vi "运维调试_采配水V2.vi"() -> ()   [LabVIEW 2016, in "PLC.lvlib"]
uses:
  PLC.lvlib
  <vilib>/Plasmionique/MB Master/MB_Master/MB_Master.lvclass
  <vilib>/Utility/miscctls.llb/LVPointTypeDef.ctl
  <vilib>/Plasmionique/MB Master/MB_Master_Serial/MB_Master_Serial.lvclass
  D:/Program Files (x86)/National Instruments/LabVIEW 2016/vi.lib/Plasmionique/MB Master/MB_Master/MB_Master.lvclass
  <vilib>/Instr/_visa.llb/VISA Configure Serial Port (Instr).vi
  <vilib>/Plasmionique/MB Master/MB Master.lvlib
panel:
  out "Registers":u16[](array[numeric])
  out "R118":i16 caption="多参数沉淀时间"
  in  "看门狗启用":bool
  out "R117":i16 caption="看门狗设置值"
  out "R33":i16 caption="看门狗计时器"
  in  "更新程序":bool
  in  "R116":i16(ring) caption="储水水体选择" items=["自来水", "采水泵"]
  out "当前启动泵号":u16(ring) items=["1号水样泵", "2号水样泵"]
  out "R113":i16 caption="储水时间设定"
  out "R25":i16
  in  "V14NC":bool
  out "R24":i16
  in  "V14NO":bool
  out "X2":bool caption="X1"
  out "采配水版本号":string
  out "R23":i16 caption="清洗频次计数"
  out "R112":i16 caption="清洗频次设定"
  out "R22":i16
  in  "V13NC":bool
  out "R111":i16 caption="排液时间"
  out "通讯故障":bool
  out "R21":i16
  in  "V13NO":bool
  out "R20":i16
  in  "M1-2":bool
  in  "潜水泵工作模式":u16(ring) items=["泵1单泵单管路", "泵2单泵单管路", "潜水泵双泵双管路", "自吸泵双泵双管路"]
  out "X11":bool caption="废液报警"
  out "X10":bool caption="自来水检测"
  out "X9":bool caption="泵2过载报警"
  out "X8":bool caption="泵1过载报警"
  out "X7":bool caption="断电检测"
  out "X6":bool caption="开门检测"
  out "X5":bool caption="烟雾检测"
  out "X4":bool caption="漏水检测"
  out "X3":bool caption="进样检测"
  out "X1":bool
  out "X0":bool caption="采样池液位开关"
  out "R109":i16 caption="配水时间"
  out "集成报警信息":string
  out "R108":i16 caption="自来水报警"
  out "R107":i16 caption="采水池液位报警设置"
  out "R106":i16 caption="进样超时设置"
  out "R105":i16 caption="二级清洗时间"
  out "R104":i16 caption="一级清洗时间"
  out "R103":i16 caption="外部管路清洗时间"
  out "R102":i16 caption="静置沉淀时间"
  out "R101":i16 caption="内部管路润洗时间"
  out "R100":i16 caption="外部管路润洗时间"
  out "R2":i16
  out "R1":i16
  out "多列列表框":i32(listbox)
  out "R19":i16
  in  "V6":bool
  out "R18":i16
  in  "V5":bool
  out "R17":i16
  in  "V4":bool
  out "R16":i16
  in  "V3":bool
  out "R15":i16
  in  "V2":bool
  out "R14":i16
  in  "M2":bool
  out "R13":i16
  in  "V1":bool
  out "R12":i16
  in  "M1-1":bool
  in  "返回":bool
  in  "参数设置":bool
  in  "单步启动":bool
  in  "启动":bool
  in  "停止":bool
  # "看门狗设置"
  # "S"
  # "S"
  # "S"
  # "S"
  # "次"
  # "次"
  # "S"
  # "S"
  # "S"
  # "S"
  # "S"
  # "S"
  # "S"
  # "S"
  # "S"
  # "S"
  # "S"
  # "单步计时："
  # "s"
  # "流程计时："
  # "s"
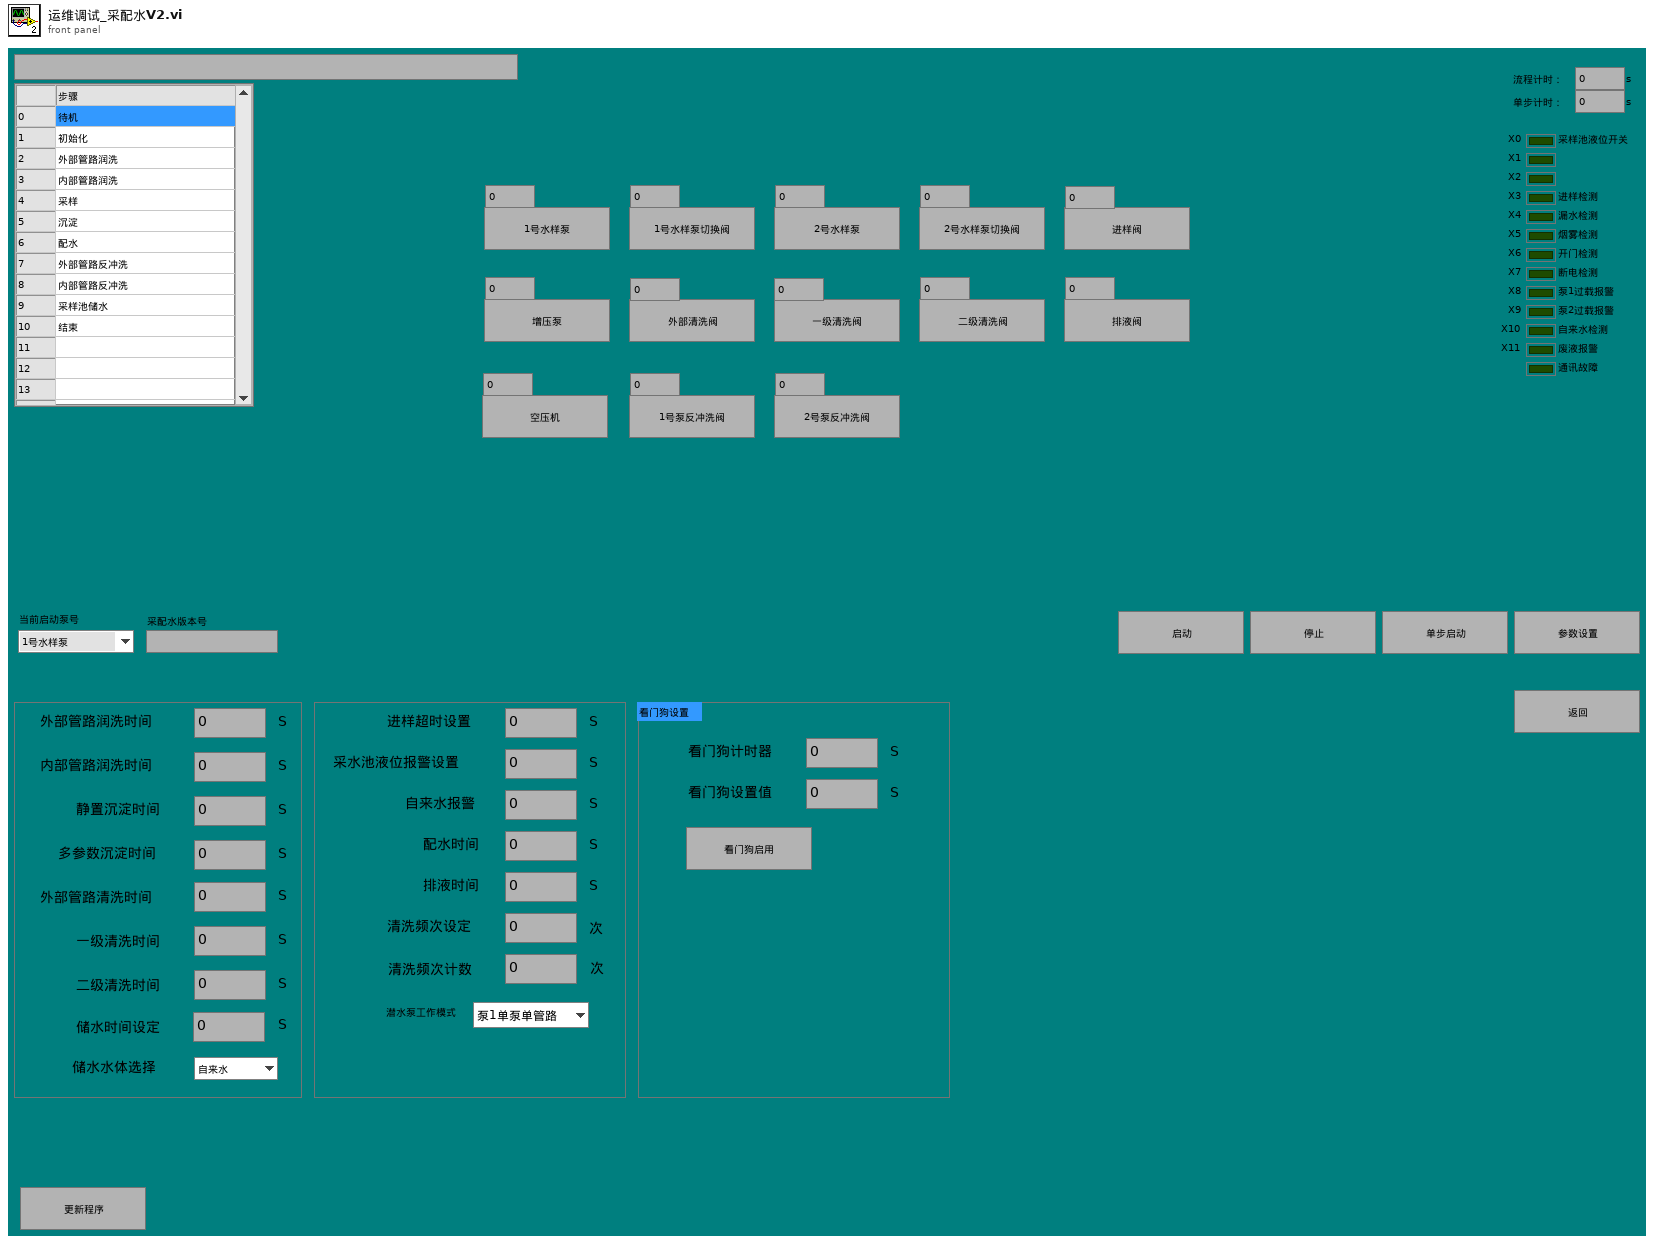
[diagram p1: front panel]
types:
  T1 = typedef "参数.ctl" = cluster{"测试模式":enum16{"水样测试", "平行样测试", "集成干预测试", "加标回收"}, "参数启用":T2}
  T2 = typedef "启动参数.ctl" = cluster{"氨氮":bool, "总磷":bool, "总氮":bool, "多参数":bool, "CODmn":bool, "CODCr":bool, "氟化物":bool, "超标留样启用":bool}
  T3 = typedef "LVPointTypeDef.ctl" = cluster{"Horizontal":i16, "Vertical":i16}
  T4 = cluster{"命令":string, "数据":cluster{"starting address":u16, "holding register value":u16}}
  T5 = cluster{"命令":string, cluster{"starting address":u16, "holding register value":u16}}
  T6 = cluster{"命令":string, "数据":cluster{"starting address":u16, "holding register values":u16[]}}
  T7 = cluster{"命令":string, "data":cluster{"starting address":u16, "coil values":bool[]}}
  T8 = cluster{"测试模式":enum16{"水样测试", "平行样测试", "集成干预测试", "加标回收"}, "参数启用":T2}
  T9 = cluster{"R0":i16, "R1":i16, "R2":i16, "R3":i16, "R4":i16, "R5":i16, "R6":i16, "R7":i16, "R8":i16, "R9":i16, "R10":i16, "R11":i16, "R12":i16, "R13":i16, "R14":i16, "R15":i16, "R16":i16, "R17":i16, "R18":i16, "R19":i16, "R20":i16, "R21":i16, "R22":i16, "R23":i16, "R24":i16, "R25":i16, "R26":i16, "R27":i16, "R28":i16, "R29":i16, "R30":i16, "R31":i16, "R32":i16, "R33":i16, "R34":i16, "R35":i16, "R36":i16, "R37":i16, "R38":i16, "R39":i16, "R40":i16, "R41":i16, "R42":i16, "R43":i16, "R44":i16, "R45":i16, "R46":i16, "R47":i16, "R48":i16, "R49":i16, "R50":i16, "R51":i16, "R52":i16, "R53":i16, "R54":i16, "R55":i16, "R56":i16, "R57":i16, "R58":i16, "R59":i16, "R60":i16, "R61":i16, "R62":i16, "R63":i16, "R64":i16, "R65":i16, "R66":i16, "R67":i16, "R68":i16, "R69":i16, "R70":i16, "R71":i16, "R72":i16, "R73":i16, "R74":i16, "R75":i16, "R76":i16, "R77":i16, "R78":i16, "R79":i16}
  T10 = cluster{"R100":i16, "R101":i16, "R102":i16, "R103":i16, "R104":i16, "R105":i16, "R106":i16, "R107":i16, "R108":i16, "R109":i16, "R110":i16, "R111":i16, "R112":i16, "R113":i16, "R114":i16, "R115":i16, "R116":i16, "R117":i16, "R118":i16, "R119":i16, "R120":i16, "R121":i16, "R122":i16, "R123":i16, "R124":i16, "R125":i16, "R126":i16, "R127":i16, "R128":i16, "R129":i16, "R130":i16, "R131":i16, "R132":i16, "R133":i16}
  T11 = cluster{"seconds since 1Jan1904":timestamp, "table输入":string, string, "table输入":string}
  T12 = cluster{"baud rate (bps)":u32, "stop bits":u16, "parity":u16, "flow control":u16, "timeout":u32, "retries":i32}
  T13 = cluster{"starting address":u16, "holding register values":u16[]}
  T14 = cluster{"starting address":u16, "holding register value":u16}
  T15 = cluster{"starting address":u16, "coil values":bool[]}
  T16 = cluster{"Registers[0]":u16, "Registers[1]":u16, "Registers[2]":u16, "Registers[3]":u16, "Registers[4]":u16, "Registers[5]":u16, "Registers[6]":u16, "Registers[7]":u16, "Registers[8]":u16, "Registers[9]":u16, "Registers[10]":u16, "Registers[11]":u16, "Registers[12]":u16, "Registers[13]":u16, "Registers[14]":u16, "Registers[15]":u16, "Registers[16]":u16, "Registers[17]":u16, "Registers[18]":u16, "Registers[19]":u16, "Registers[20]":u16, "Registers[21]":u16, "Registers[22]":u16, "Registers[23]":u16, "Registers[24]":u16, "Registers[25]":u16, "Registers[26]":u16, "Registers[27]":u16, "Registers[28]":u16, "Registers[29]":u16, "Registers[30]":u16, "Registers[31]":u16, "Registers[32]":u16, "Registers[33]":u16, "Registers[34]":u16, "Registers[35]":u16, "Registers[36]":u16, "Registers[37]":u16, "Registers[38]":u16, "Registers[39]":u16, "Registers[40]":u16, "Registers[41]":u16, "Registers[42]":u16, "Registers[43]":u16, "Registers[44]":u16, "Registers[45]":u16, "Registers[46]":u16, "Registers[47]":u16, "Registers[48]":u16, "Registers[49]":u16, "Registers[50]":u16, "Registers[51]":u16, "Registers[52]":u16, "Registers[53]":u16, "Registers[54]":u16, "Registers[55]":u16, "Registers[56]":u16, "Registers[57]":u16, "Registers[58]":u16, "Registers[59]":u16, "Registers[60]":u16, "Registers[61]":u16, "Registers[62]":u16, "Registers[63]":u16, "Registers[64]":u16, "Registers[65]":u16, "Registers[66]":u16, "Registers[67]":u16, "Registers[68]":u16, "Registers[69]":u16, "Registers[70]":u16, "Registers[71]":u16, "Registers[72]":u16, "Registers[73]":u16, "Registers[74]":u16, "Registers[75]":u16, "Registers[76]":u16, "Registers[77]":u16, "Registers[78]":u16, "Registers[79]":u16}
  T17 = cluster{"Registers[0]":u16, "Registers[1]":u16, "Registers[2]":u16, "Registers[3]":u16, "Registers[4]":u16, "Registers[5]":u16}
  T18 = cluster{"Registers[0]":u16, "Registers[1]":u16, "Registers[2]":u16, "Registers[3]":u16, "Registers[4]":u16, "Registers[5]":u16, "Registers[6]":u16, "Registers[7]":u16, "Registers[8]":u16, "Registers[9]":u16, "Registers[10]":u16, "Registers[11]":u16, "Registers[12]":u16, "Registers[13]":u16, "Registers[14]":u16, "Registers[15]":u16, "Registers[16]":u16, "Registers[17]":u16, "Registers[18]":u16, "Registers[19]":u16, "Registers[20]":u16, "Registers[21]":u16, "Registers[22]":u16, "Registers[23]":u16, "Registers[24]":u16, "Registers[25]":u16, "Registers[26]":u16, "Registers[27]":u16, "Registers[28]":u16, "Registers[29]":u16, "Registers[30]":u16, "Registers[31]":u16, "Registers[32]":u16, "Registers[33]":u16}
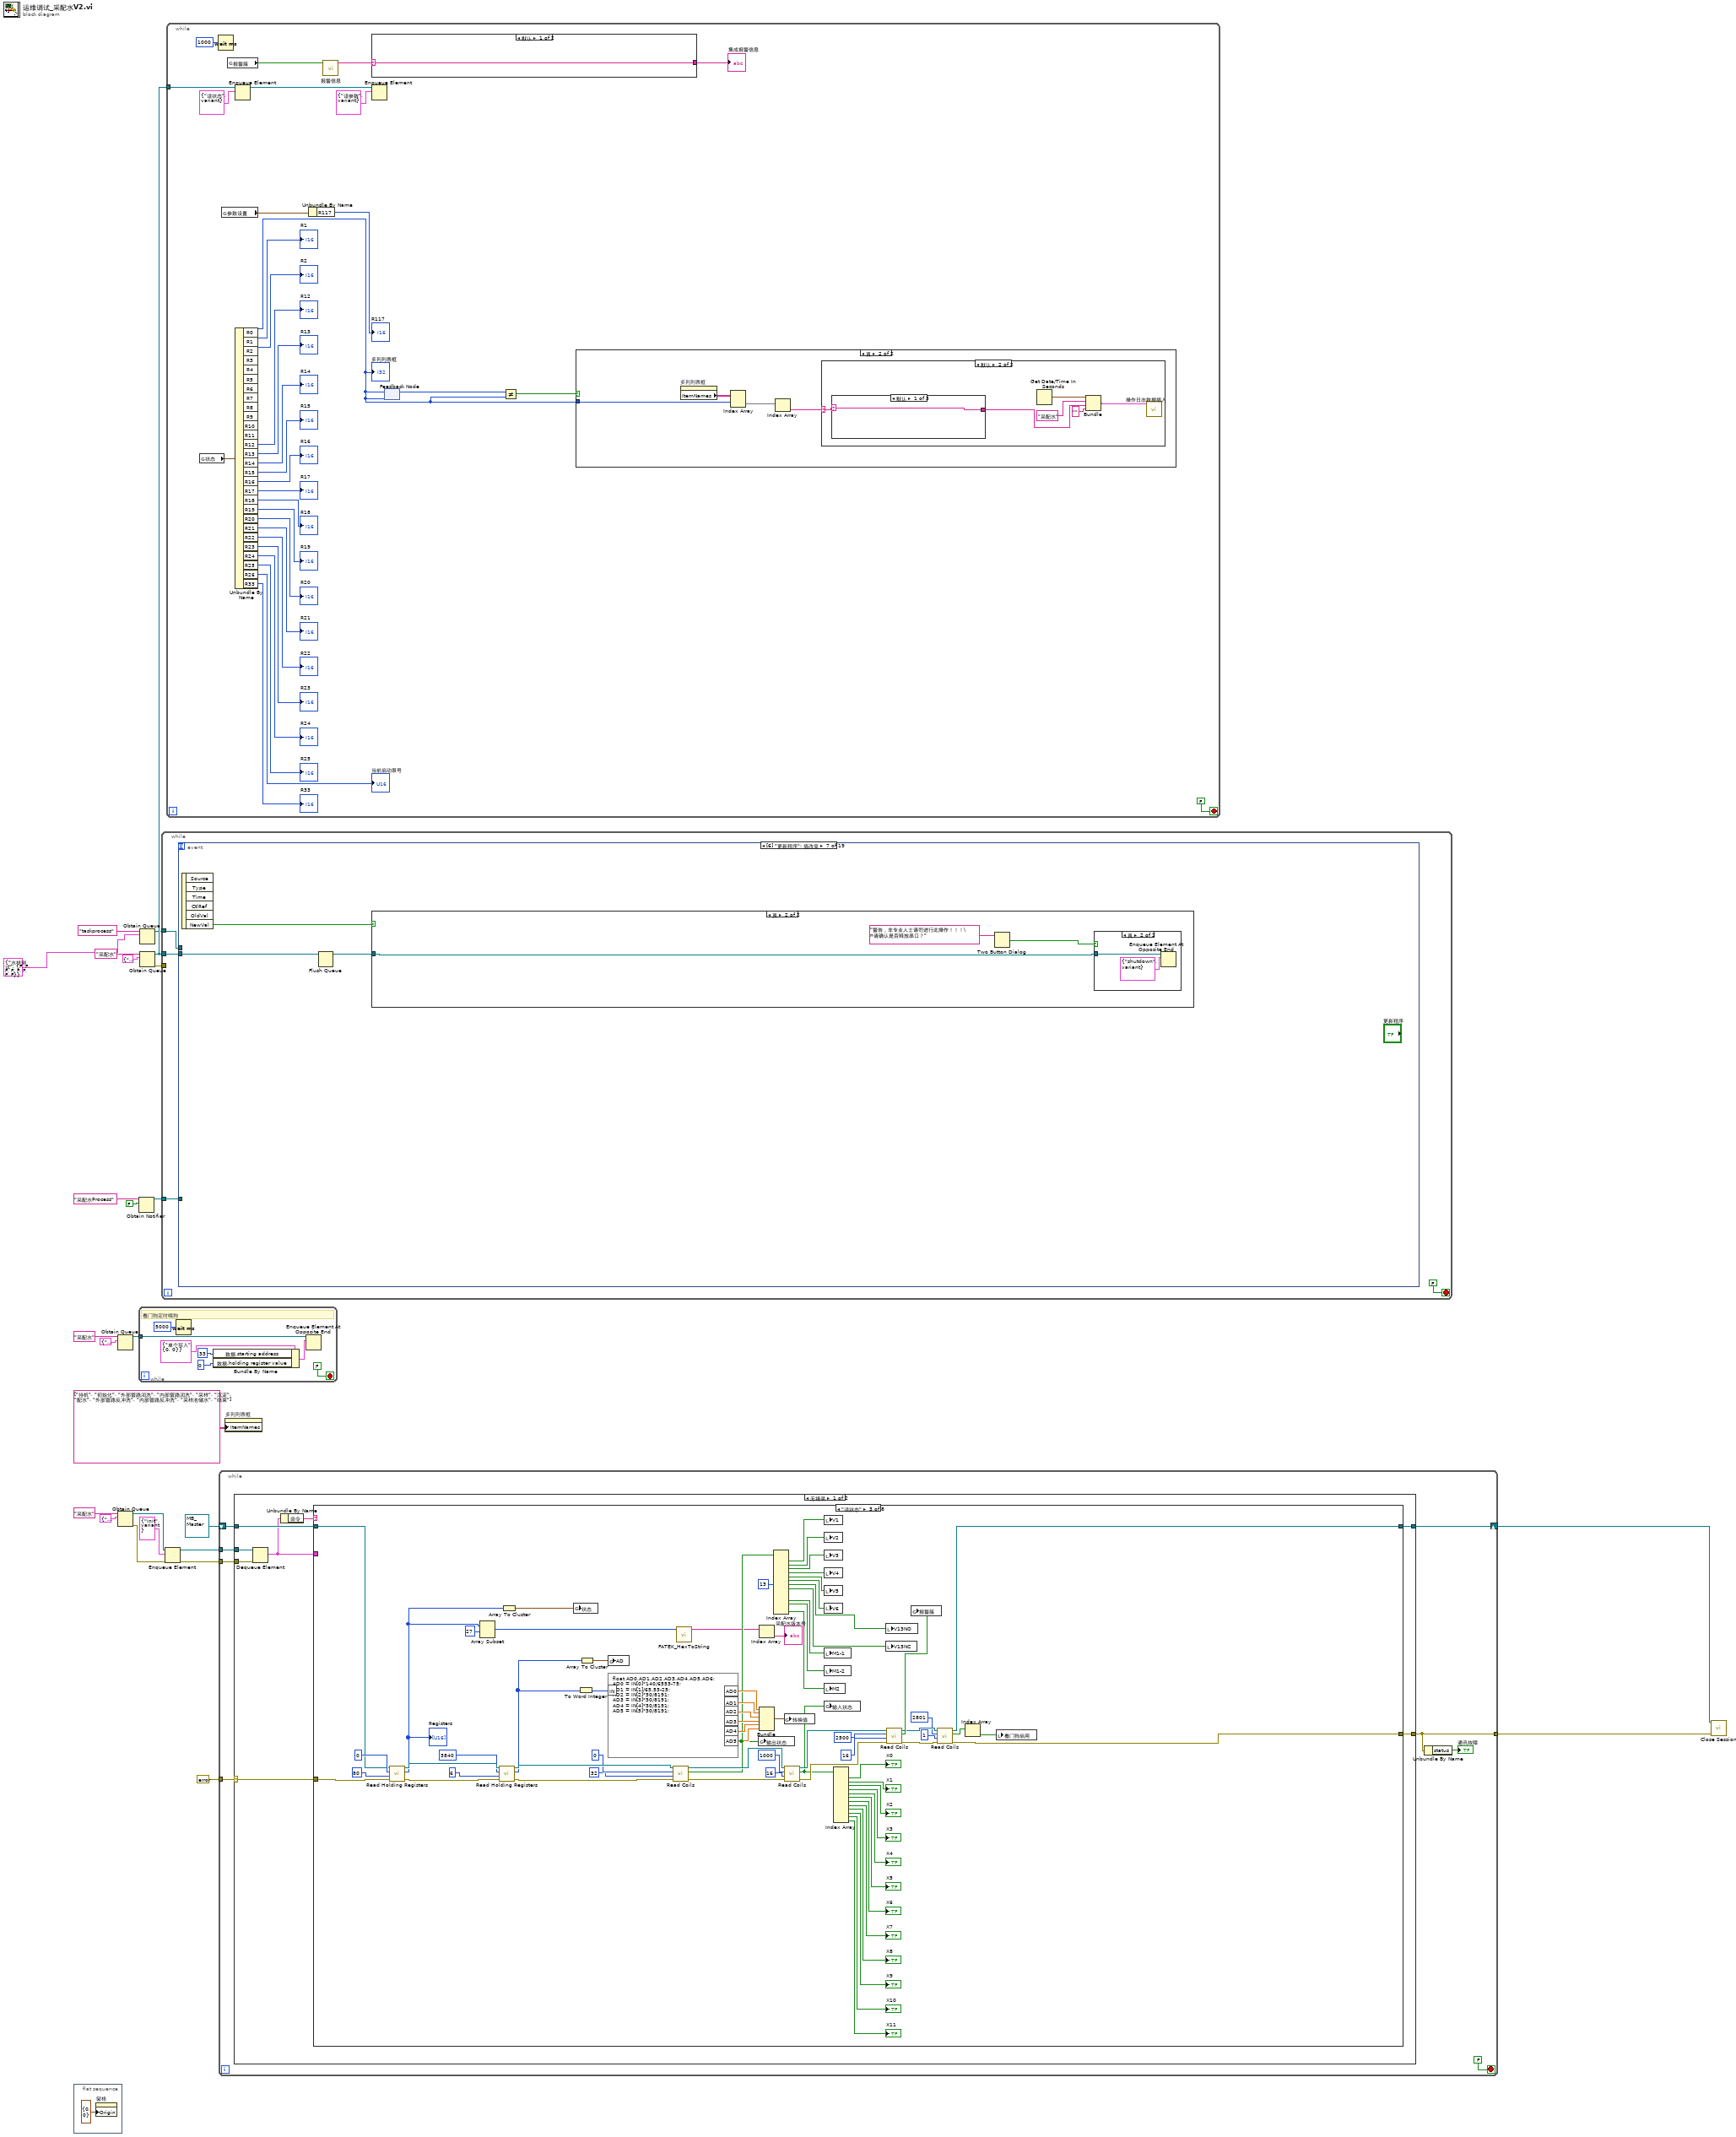
[diagram p0: block diagram]
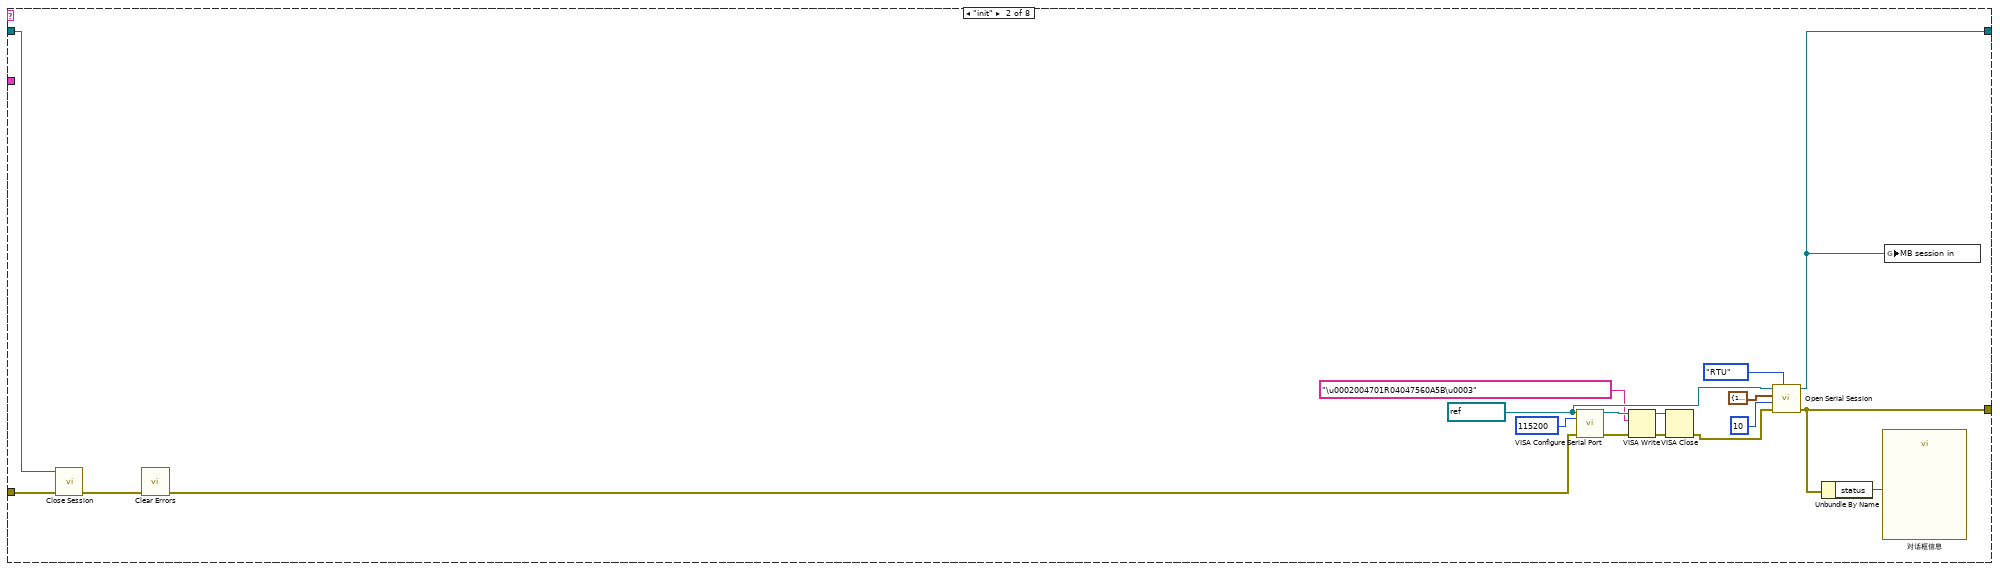
[diagram p3: hidden frame]
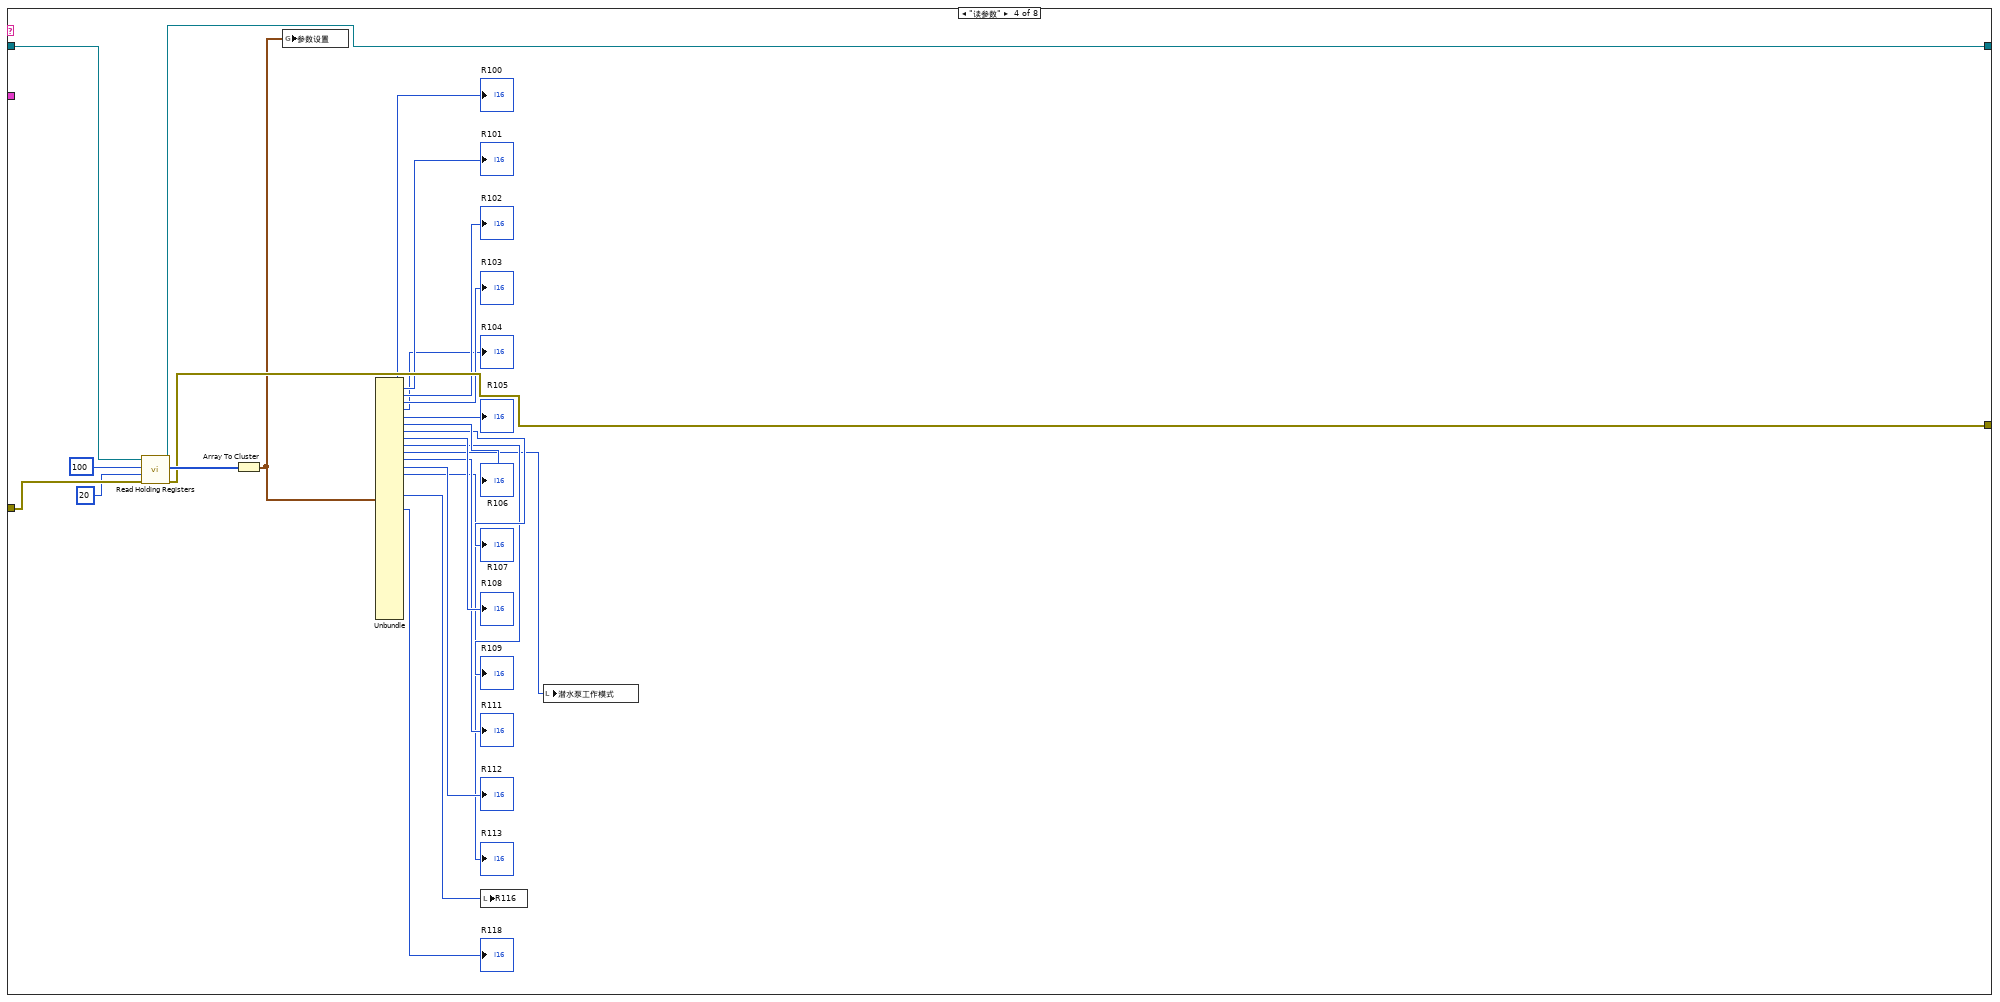
[diagram p4: hidden frame]
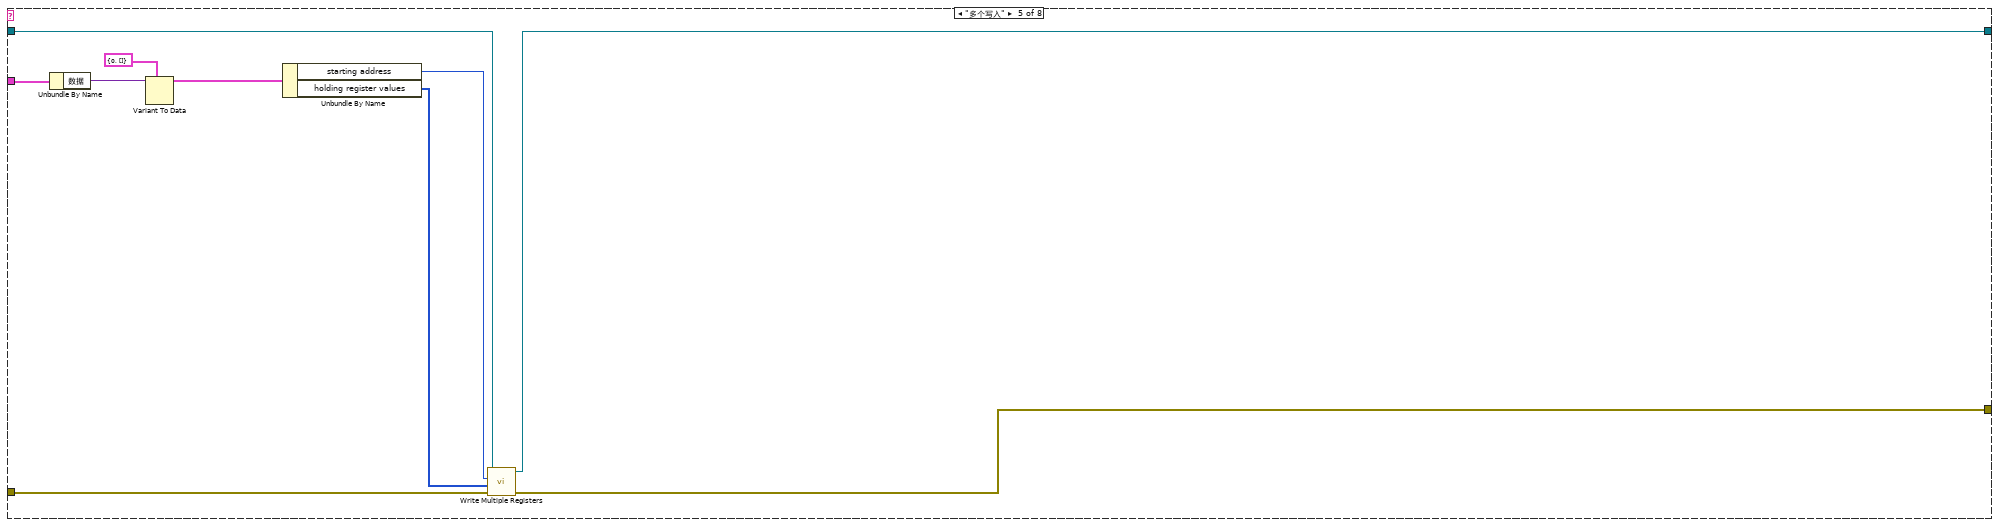
[diagram p5: hidden frame]
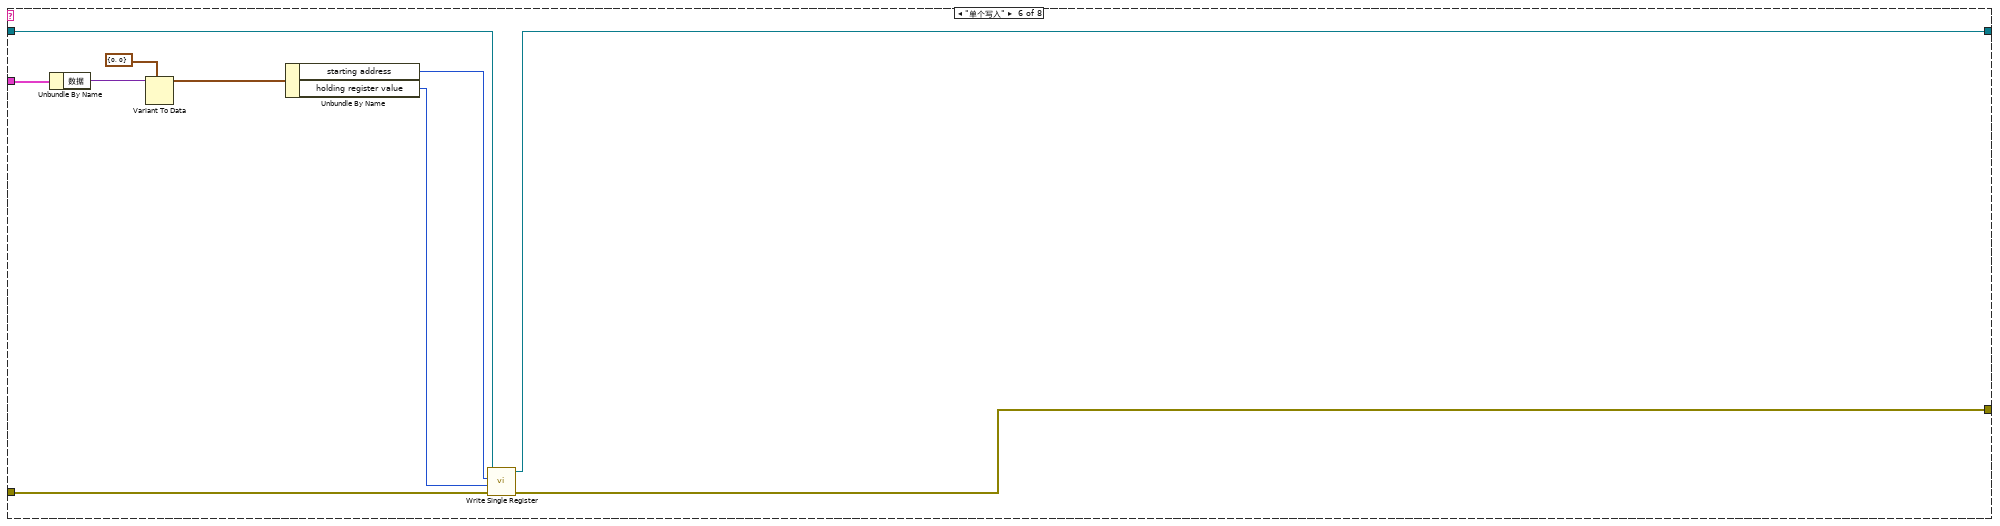
[diagram p6: hidden frame]
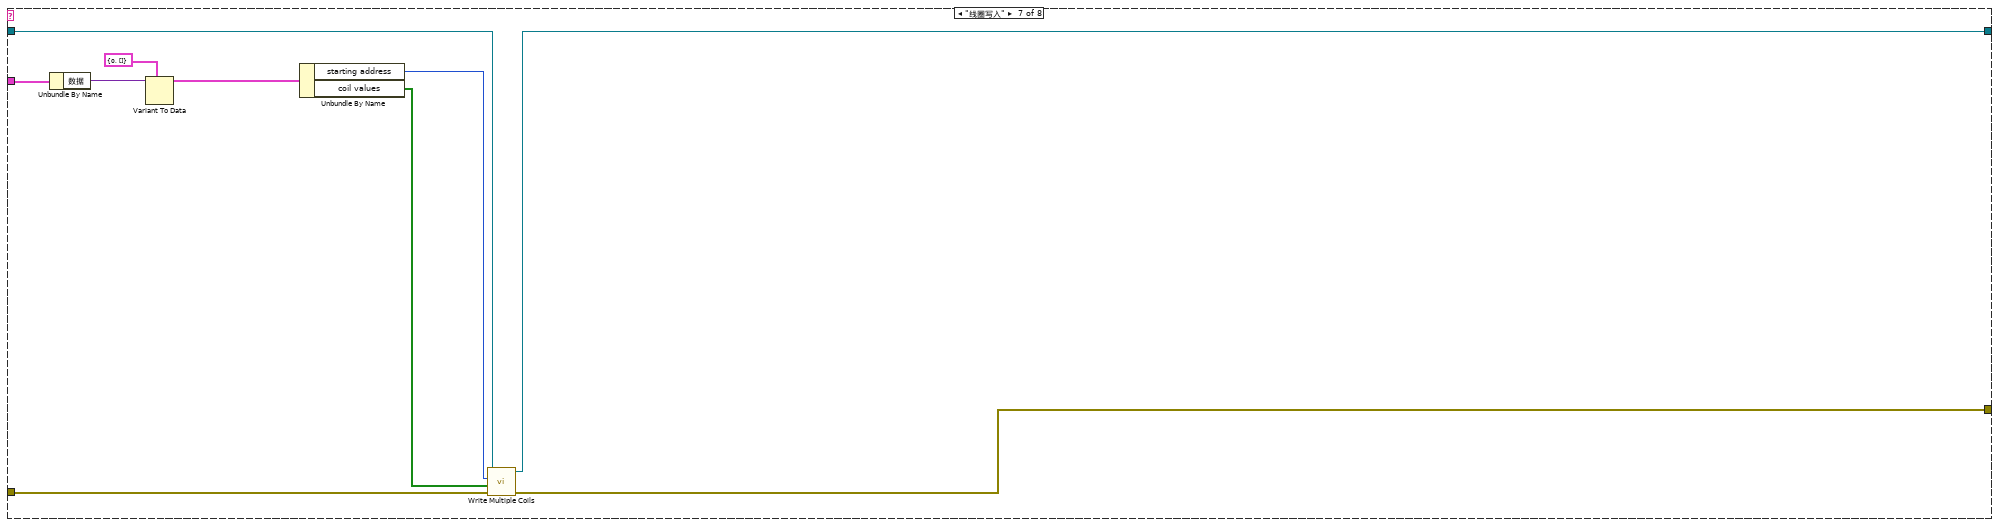
[diagram p7: hidden frame]
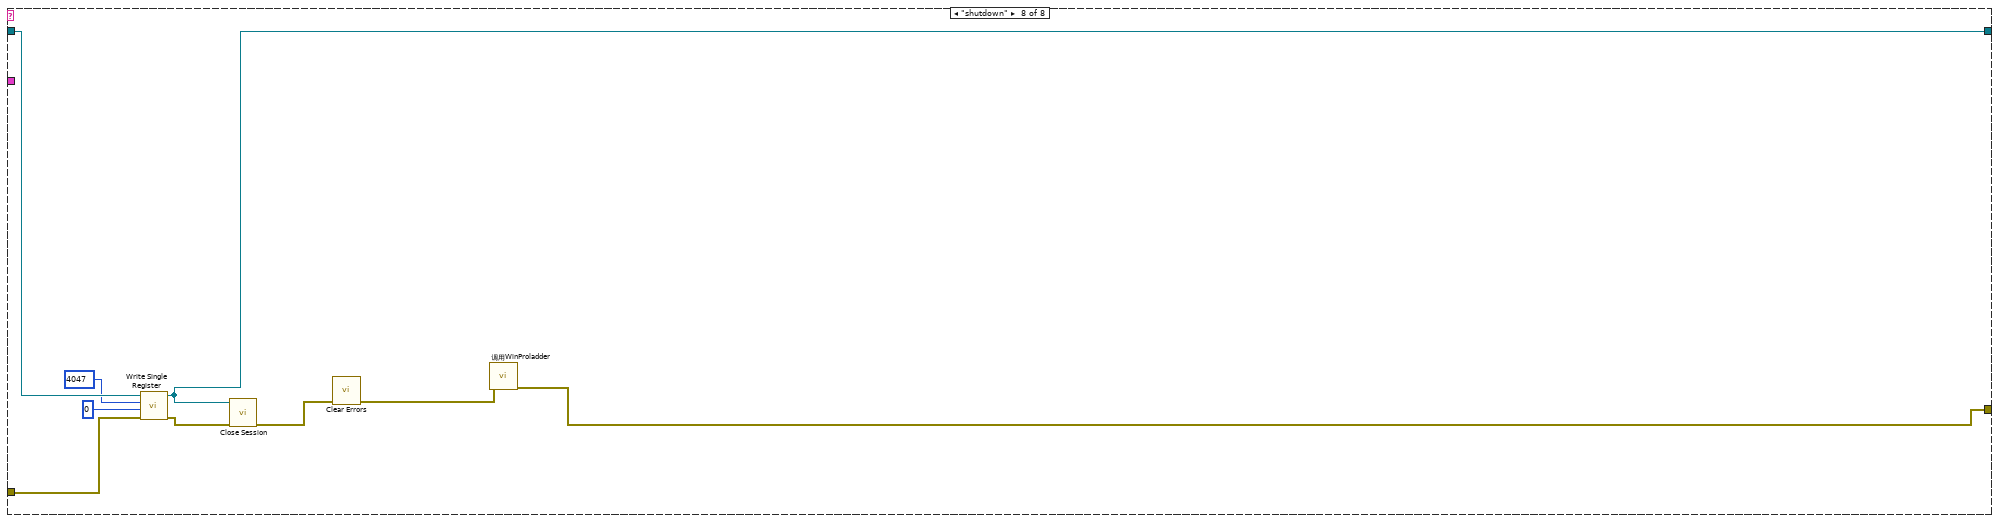
[diagram p8: hidden frame]
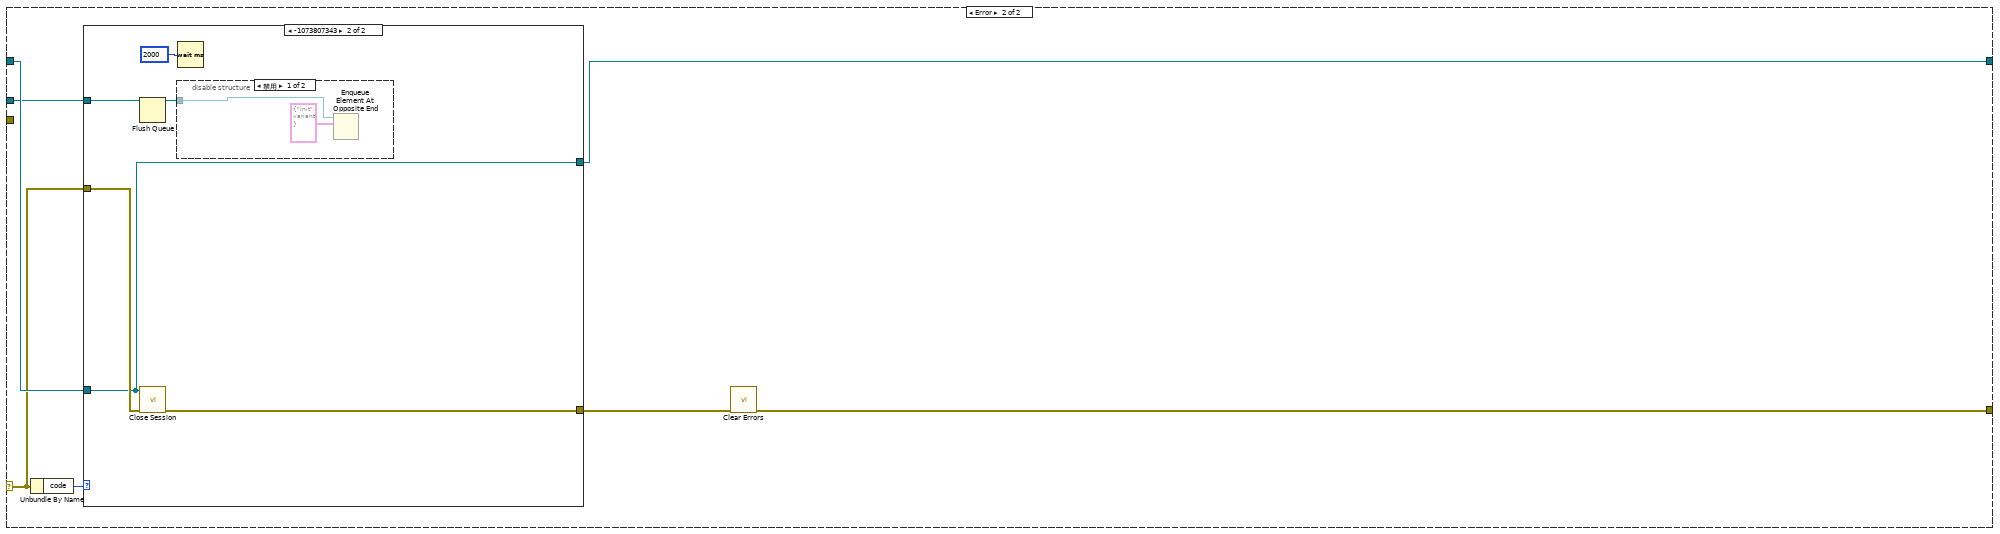
[diagram p9: hidden frame]
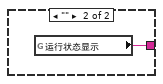
[diagram p12: hidden frame]
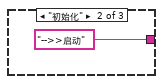
[diagram p15: hidden frame]
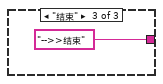
[diagram p16: hidden frame]
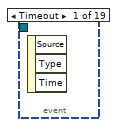
[diagram p17: hidden frame]
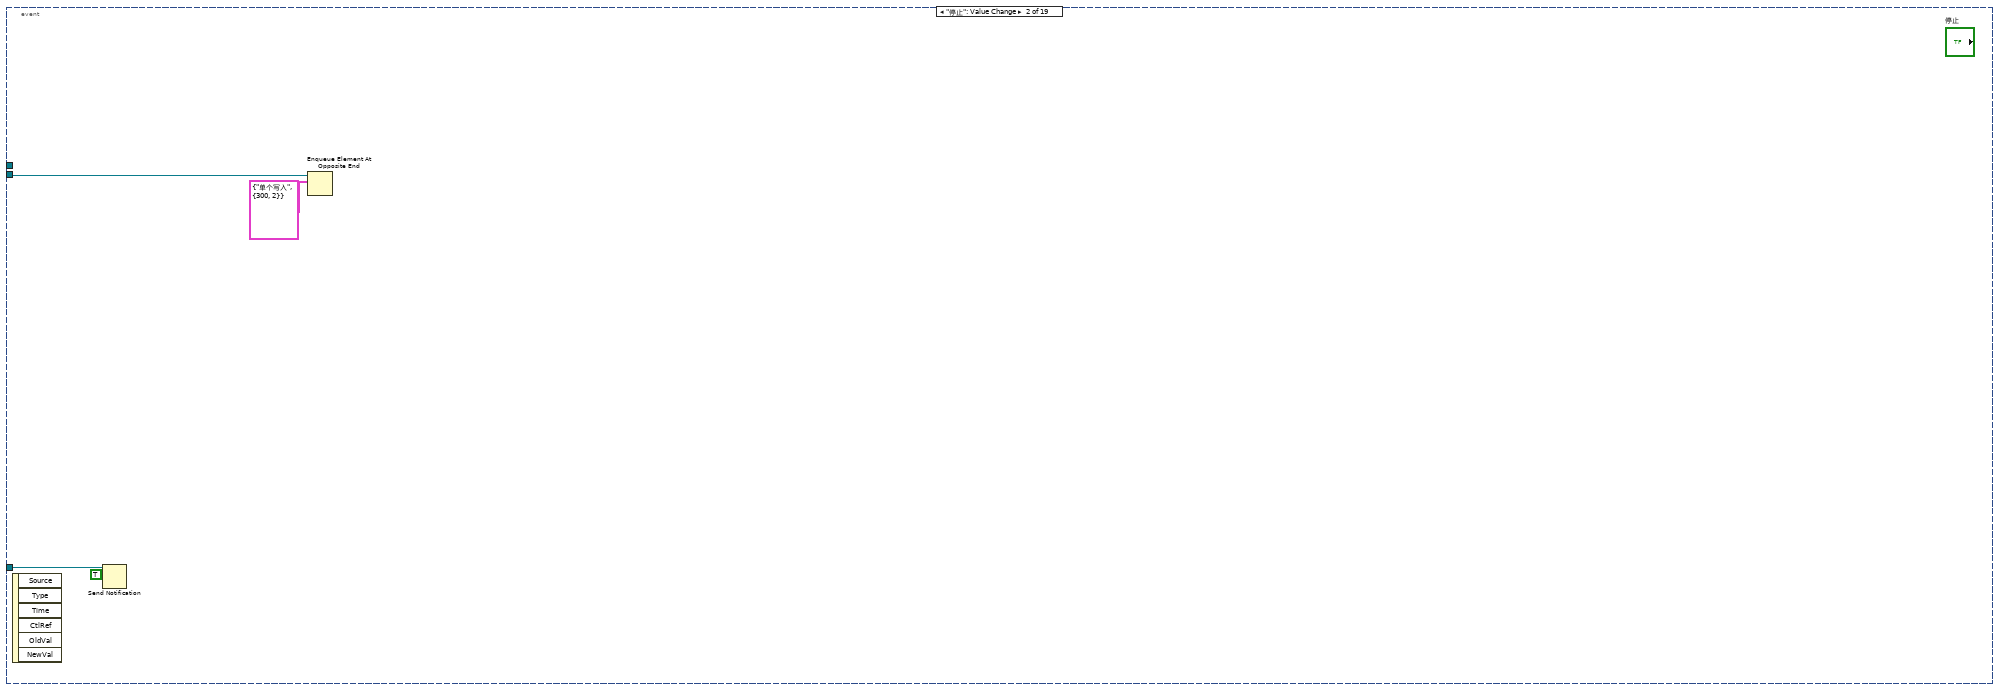
[diagram p18: hidden frame]
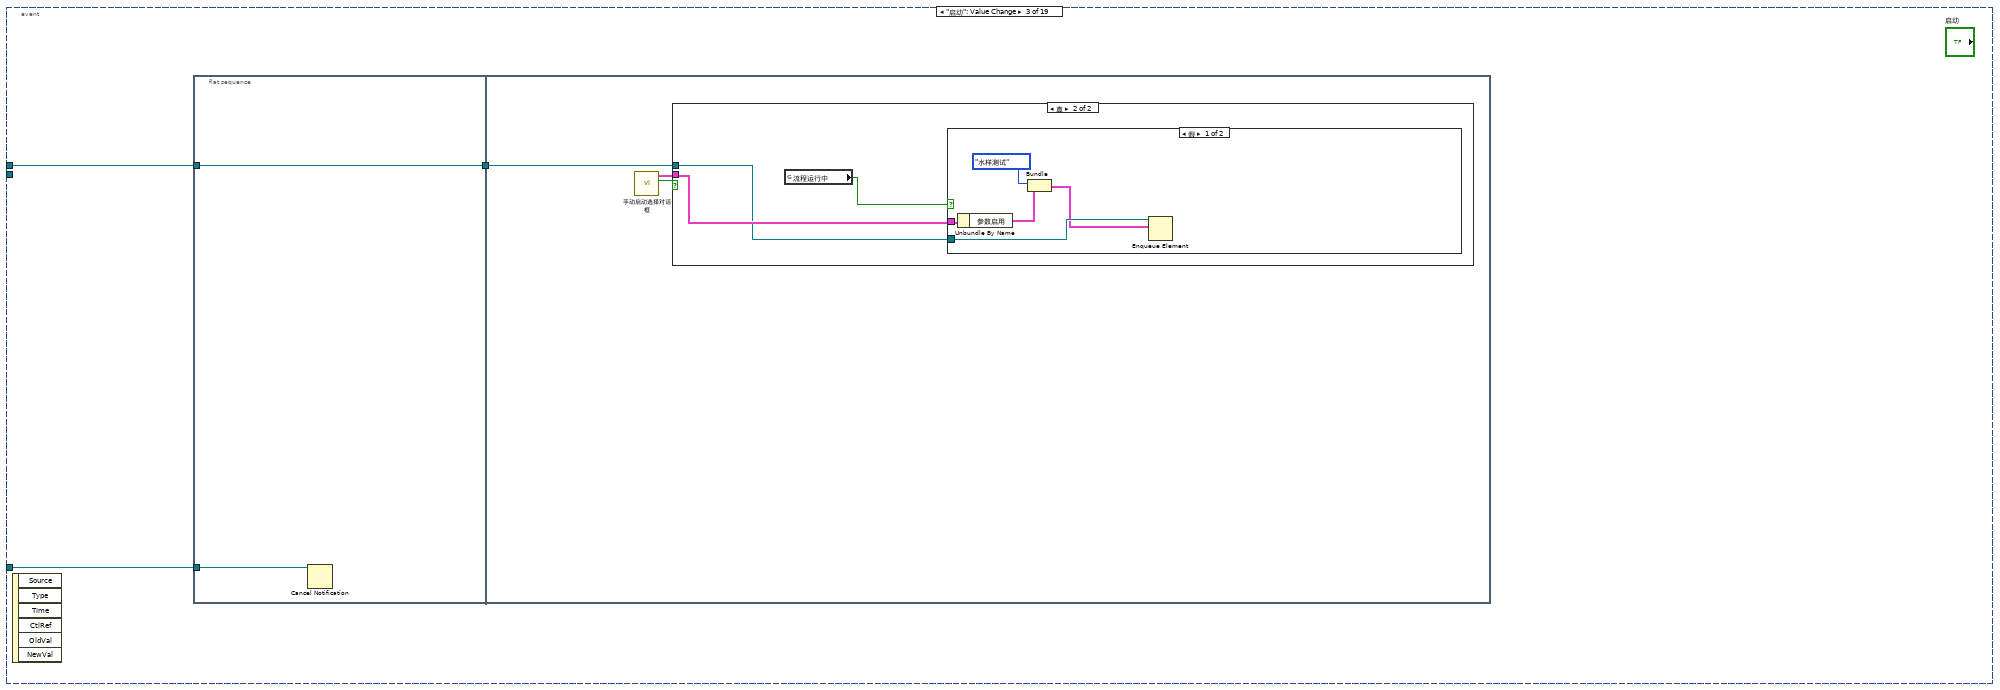
[diagram p19: hidden frame]
diagram:
  n1 = flat-sequence {
    frame #0 {
      n2 = property on="窗格" class="Pane"("Origin"=T3 {"Horizontal"=0, "Vertical"=0} ("原点")) -> ()  [unwired: 2 in, 2 out]
    }
  }
  n3 = Obtain Queue(name (unnamed)="采配水" ("名称（未命名）"), element data type=cluster{"命令":string, "数据":variant} {"命令"="", "数据"=variant}) -> (queue out=w4:refnum<queue>)  [unwired: 3 in, 2 out]
  n4 = Obtain Queue(name (unnamed)="采配水" ("名称（未命名）"), element data type=cluster{"命令":string, "数据":variant} {"命令"="", "数据"=variant}) -> (queue out=w15:refnum<queue>, error out=w14:errorcluster)  [unwired: 3 in, 1 out]
  n5 = Obtain Notifier(name (unnamed)="采配水Process" ("名称（未命名）"), notification data type=FALSE) -> (notifier out=w18:refnum<notifier>)  [unwired: 2 in, 2 out]
  n6 = while {
    tunnel: w4 -> [w29]
    stop <- FALSE stop-if-true
    # "看门狗定时喂狗"
    n7 = Wait (ms)(milliseconds to wait=u32 5000 ("等待时间（毫秒）")) -> ()  [unwired: 1 out]
    n8 = Bundle By Name(cluster=T4 {"命令"="单个写入", "数据"={"starting address"=0, "holding register value"=0}} ("元素"), "数据.starting address"=u16 33, "数据.holding register value"=u16 0) -> (w30:T4)
    n9 = Enqueue Element At Opposite End(queue=w29, element=w30) -> ()  [unwired: 2 in, 3 out]
  }
  n10 = Obtain Queue(name (unnamed)="taskprocess" ("名称（未命名）"), element data type=T1 {"测试模式"=enum."水样测试", "参数启用"={"氨氮"=FALSE, "总磷"=FALSE, "总氮"=FALSE, "多参数"=FALSE, "CODmn"=FALSE, "CODCr"=FALSE, "氟化物"=FALSE, "超标留样启用"=FALSE}} ("参数")) -> (queue out=w2:refnum<queue>)  [unwired: 3 in, 2 out]
  n11 = Obtain Queue(name (unnamed)="采配水" ("名称（未命名）"), element data type=cluster{"命令":string, "数据":variant} {"命令"="", "数据"=variant}) -> (queue out=w22:refnum<queue>, error out=w23:errorcluster)  [unwired: 3 in, 1 out]
  n12 = while {
    tunnel: w22 -> [w36]
    tunnel: w23 -> [_]
    tunnel: w18 -> [w35]
    tunnel: w2 -> [w34]
    stop <- FALSE stop-if-true
    n13 = event shown="[6] \"更新程序\": 值改变" {
      selector: _ -> [_ _ _ _ _ _ _ _ _ _ _ _ _ _ _ _ _ _ _]
      dyn-events: _ -> [_ _ _ _ _ _ _ _ _ _ _ _ _ _ _ _ _ _ _]
      timeout: _ -> [_ _ _ _ _ _ _ _ _ _ _ _ _ _ _ _ _ _ _]
      tunnel: w36 -> [_ w40 _ w62 w81 w86 w92 w103 _ _ _ _ w131 w133 w138 w143 w148 w153 w158]
      tunnel: w35 -> [_ w39 w44 _ _ _ _ _ _ _ _ _ _ _ _ _ _ _ _]
      tunnel: w34 -> [_ _ w42 _ _ _ _ _ _ _ _ _ _ _ _ _ _ _ _]
      event Timeout {
        n14 = event-data() -> ()  [unwired: 1 in, 3 out]
      }
      event "停止": Value Change {
        n15 = event-data() -> ()  [unwired: 1 in, 6 out]
        n16 = Send Notification(notification=TRUE ("通知"), notifier=w39) -> ()  [unwired: 1 in, 2 out]
        n17 = Enqueue Element At Opposite End(queue=w40, element=T5 {"命令"="单个写入", {"starting address"=300, "holding register value"=2}} ("元素")) -> ()  [unwired: 2 in, 3 out]
      }
      event "启动": Value Change {
        n18 = event-data() -> ()  [unwired: 1 in, 6 out]
        n19 = flat-sequence {
          tunnel: w44 -> [w46]
          tunnel: [w45] -> w43
          tunnel: w42 -> [w45]
          tunnel: w43 -> [w47]
          frame #0 {
            n20 = Cancel Notification(0:w46) -> ()  [unwired: 1 in, 3 out]
          }
          frame #1 {
            n21 = call "手动启动选择对话框.vi"() -> ("确定"=w49:bool, "输出簇"=w48:cluster{"参数启用":T2})  [unwired: 10 in]
            n22 = case shown="真" w49 {
              tunnel: w48 -> [_ w51]
              tunnel: w47 -> [_ w50]
              frame False {
              }
              frame True {
                n23 = global read "采配水全局变量.vi" "流程运行中"() -> (w52:bool)
                n24 = case shown="假" w52 {
                  tunnel: w51 -> [w55 _]
                  tunnel: w50 -> [w57 _]
                  frame False {
                    n25 = Unbundle By Name(w55) -> ("参数启用"=w54:T2)
                    n26 = Bundle("测试模式"=enum16{"水样测试", "平行样测试", "集成干预测试", "加标回收"}."水样测试", "参数启用"=w54) -> (w53:T8)  [unwired: 1 in]
                    n27 = Enqueue Element(queue=w57, element=w53) -> ()  [unwired: 2 in, 3 out]
                  }
                  frame True {
                    n28 = One Button Dialog(message="流程已启动，无需重复启动！" ("消息")) -> ()  [unwired: 1 in, 1 out]
                  }
                }
              }
            }
          }
        }
      }
      event "单步启动": Value Change {
        n29 = event-data() -> ()  [unwired: 1 in, 6 out]
        n30 = call "单步启动对话框.vi"() -> ("单步启动步骤输出"=w59:u16)  [unwired: 11 in]
        n31 = Bundle By Name(cluster=T4 {"命令"="单个写入", "数据"={"starting address"=301, "holding register value"=0}} ("元素"), "数据.holding register value"=w59) -> (w60:T4)
        n32 = Enqueue Element At Opposite End(queue=w62, element=w60) -> ()  [unwired: 2 in, 3 out]
      }
      event "R100", "R101", "R102", "R103", "R104", "R105", "R106", "R107", "R108", "R109", "潜水泵工作模式", "R111", "R112", "R113": Value Change {
        n33 = event-data() -> ()  [unwired: 1 in, 6 out]
        n34 = local read "R100"() -> (w76:i16)
        n35 = local read "R101"() -> (w75:i16)
        n36 = local read "R102"() -> (w74:i16)
        n37 = local read "R103"() -> (w73:i16)
        n38 = local read "R104"() -> (w72:i16)
        n39 = local read "R105"() -> (w71:i16)
        n40 = local read "R106"() -> (w70:i16)
        n41 = local read "R107"() -> (w69:i16)
        n42 = local read "R108"() -> (w68:i16)
        n43 = local read "R109"() -> (w67:i16)
        n44 = local read "R111"() -> (w65:i16)
        n45 = local read "R112"() -> (w64:i16)
        n46 = local read "R113"() -> (w63:i16)
        n47 = Build Array(w76, w75, w74, w73, w72, w71, w70, w69, w68, w67, "潜水泵工作模式", w65, w64, w63) -> (w77:u16[])
        n48 = Bundle By Name(cluster=T6 {"命令"="多个写入", "数据"={"starting address"=0, "holding register values"=[]}} ("元素"), "数据.starting address"=u16 100, "数据.holding register values"=w77) -> (w78:T6)
        n49 = Enqueue Element At Opposite End(queue=w81, element=w78) -> ()  [unwired: 2 in, 3 out]
      }
      event "R116", "R117", "R118": Value Change {
        n50 = event-data() -> ()  [unwired: 1 in, 6 out]
        n51 = local read "R117"() -> (w83:i16)
        n52 = local read "R118"() -> (w82:i16)
        n53 = Build Array("R116", w83, w82) -> (w85:i16[])
        n54 = Bundle By Name(cluster=T6 {"命令"="多个写入", "数据"={"starting address"=0, "holding register values"=[]}} ("元素"), "数据.starting address"=u16 116, "数据.holding register values"=w85) -> (w87:T6)
        n55 = Enqueue Element At Opposite End(queue=w86, element=w87) -> ()  [unwired: 2 in, 3 out]
      }
      event "更新程序": Value Change {
        n56 = event-data() -> ("NewVal"=w91:bool)  [unwired: 1 in, 5 out]
        n57 = Flush Queue(queue=w92) -> (queue out=w90:refnum<queue>)  [unwired: 1 in, 2 out]
        n58 = case shown="真" w91 {
          tunnel: w90 -> [w93 w97]
          frame False {
            n59 = Enqueue Element At Opposite End(queue=w93, element=cluster{"命令":string, "数据":variant} {"命令"="init", "数据"=variant} ("元素")) -> ()  [unwired: 2 in, 3 out]
          }
          frame True {
            n60 = Two Button Dialog(message="警告，非专业人士请勿进行此操作！！！\n请确认是否释放串口？" ("消息")) -> (T button?=w95:bool)  [unwired: 2 in]
            n61 = case shown="真" w95 {
              tunnel: w97 -> [_ w100]
              frame False {
                n62 = local write "更新程序"(FALSE ("下载模式")) -> ()
              }
              frame True {
                n63 = Enqueue Element At Opposite End(queue=w100, element=cluster{"命令":string, "数据":variant} {"命令"="shutdown", "数据"=variant} ("元素")) -> ()  [unwired: 2 in, 3 out]
              }
            }
          }
        }
      }
      event "R23": Value Change {
        n64 = event-data() -> ()  [unwired: 1 in, 6 out]
        n65 = local read "R23"() -> (w102:i16)
        n66 = Build Array(w102) -> (w101:i16[])
        n67 = Bundle By Name(cluster=T6 {"命令"="多个写入", "数据"={"starting address"=0, "holding register values"=[]}} ("元素"), "数据.starting address"=u16 23, "数据.holding register values"=w101) -> (w104:T6)
        n68 = Enqueue Element At Opposite End(queue=w103, element=w104) -> ()  [unwired: 2 in, 3 out]
      }
      event "R23": Mouse Down {
        n69 = event-data() -> ("CtlRef"=w109:refnum<vi>)  [unwired: 1 in, 7 out]
        n70 = Two Button Dialog(message="请确认是否更改，更改后将影响实际清洗频次" ("消息")) -> (T button?=w108:bool)  [unwired: 2 in]
        n71 = case shown="真" w108 {
          tunnel: w109 -> [_ w110]
          frame False {
          }
          frame True {
            n72 = property class="DigNum (严格)"(reference=w110) -> (reference out=w112:refnum<vi>, "Value"=w113:i16)  [unwired: 1 in, 1 out]
            n73 = call "数字键盘.vi"("OldNumber"=w113) -> ("NewNumber"=w111:sgl)
            n74 = property class="DigNum (严格)"(reference=w112, "Val(Sgnl)"=w111) -> ()  [unwired: 1 in, 2 out]
          }
        }
      }
      event "R100", "R101", "R102", "R103", "R104", "R105", "R106", "R107", "R108", "R109", "R111", "R112", "R113", "R117", "R118": Mouse Down {
        n75 = event-data() -> ("CtlRef"=w117:refnum<vi>)  [unwired: 1 in, 7 out]
        n76 = property class="DigNum (严格)"(reference=w117) -> (reference out=w115:refnum<vi>, "Value"=w116:i16)  [unwired: 1 in, 1 out]
        n77 = call "数字键盘.vi"("OldNumber"=w116) -> ("NewNumber"=w114:sgl)
        n78 = property class="DigNum (严格)"(reference=w115, "Val(Sgnl)"=w114) -> ()  [unwired: 1 in, 2 out]
      }
      event "参数设置": Value Change {
        n79 = event-data() -> ()  [unwired: 1 in, 6 out]
        n80 = property on="窗格" class="Pane"("Origin"=T3 {"Horizontal"=0, "Vertical"=628} ("原点")) -> ()  [unwired: 2 in, 2 out]
      }
      event "返回": Value Change {
        n81 = event-data() -> ()  [unwired: 1 in, 6 out]
        n82 = property on="窗格" class="Pane"("Origin"=T3 {"Horizontal"=0, "Vertical"=0} ("原点")) -> ()  [unwired: 2 in, 2 out]
      }
      event "M1-1", "V1", "M2", "V2", "V3", "V4", "V5", "V6": Value Change {
        n83 = event-data() -> ()  [unwired: 1 in, 6 out]
        n84 = Build Array("M1-1", "V1", "M2", "V2", "V3", "V4", "V5", "V6") -> (w120:bool[])
        n85 = Bundle By Name(cluster=T7 {"命令"="线圈写入", "data"={"starting address"=2400, "coil values"=[]}} ("元素"), "data.coil values"=w120) -> (w121:T7)
        n86 = Enqueue Element(queue=w131, element=w121) -> ()  [unwired: 2 in, 3 out]
      }
      event "M1-2": Value Change {
        n87 = event-data() -> ()  [unwired: 1 in, 6 out]
        n88 = Build Array("M1-2") -> (w134:bool[])
        n89 = Bundle By Name(cluster=T7 {"命令"="线圈写入", "data"={"starting address"=2413, "coil values"=[]}} ("元素"), "data.coil values"=w134) -> (w135:T7)
        n90 = Enqueue Element(queue=w133, element=w135) -> ()  [unwired: 2 in, 3 out]
      }
      event "看门狗启用": Value Change {
        n91 = event-data() -> ()  [unwired: 1 in, 6 out]
        n92 = Build Array("看门狗启用") -> (w139:bool[])
        n93 = Bundle By Name(cluster=T7 {"命令"="线圈写入", "data"={"starting address"=2801, "coil values"=[]}} ("元素"), "data.coil values"=w139) -> (w140:T7)
        n94 = Enqueue Element(queue=w138, element=w140) -> ()  [unwired: 2 in, 3 out]
      }
      event "V13NO": Value Change {
        n95 = event-data() -> ()  [unwired: 1 in, 6 out]
        n96 = Build Array("V13NO") -> (w144:bool[])
        n97 = Bundle By Name(cluster=T7 {"命令"="线圈写入", "data"={"starting address"=2414, "coil values"=[]}} ("元素"), "data.coil values"=w144) -> (w145:T7)
        n98 = Enqueue Element(queue=w143, element=w145) -> ()  [unwired: 2 in, 3 out]
      }
      event "V13NC": Value Change {
        n99 = event-data() -> ()  [unwired: 1 in, 6 out]
        n100 = Build Array("V13NC") -> (w149:bool[])
        n101 = Bundle By Name(cluster=T7 {"命令"="线圈写入", "data"={"starting address"=2415, "coil values"=[]}} ("元素"), "data.coil values"=w149) -> (w150:T7)
        n102 = Enqueue Element(queue=w148, element=w150) -> ()  [unwired: 2 in, 3 out]
      }
      event "V14NO": Value Change {
        n103 = event-data() -> ()  [unwired: 1 in, 6 out]
        n104 = Build Array("V14NO") -> (w154:bool[])
        n105 = Bundle By Name(cluster=T7 {"命令"="线圈写入", "data"={"starting address"=2408, "coil values"=[]}} ("元素"), "data.coil values"=w154) -> (w155:T7)
        n106 = Enqueue Element(queue=w153, element=w155) -> ()  [unwired: 2 in, 3 out]
      }
      event "V14NC": Value Change {
        n107 = event-data() -> ()  [unwired: 1 in, 6 out]
        n108 = Build Array("V14NC") -> (w159:bool[])
        n109 = Bundle By Name(cluster=T7 {"命令"="线圈写入", "data"={"starting address"=2409, "coil values"=[]}} ("元素"), "data.coil values"=w159) -> (w160:T7)
        n110 = Enqueue Element(queue=w158, element=w160) -> ()  [unwired: 2 in, 3 out]
      }
    }
  }
  n111 = Enqueue Element(queue=w15, element=cluster{"命令":string, "数据":variant} {"命令"="init", "数据"=variant} ("元素"), error in (no error)=w14) -> (queue out=w10:refnum<queue>, error out=w12:errorcluster)  [unwired: 1 in, 1 out]
  n112 = while {
    tunnel: w22 -> [w193]
    stop <- FALSE stop-if-true
    n113 = global read "采配水全局变量.vi" "状态"() -> (w191:T9)
    n114 = Wait (ms)(milliseconds to wait=u32 1000 ("等待时间（毫秒）")) -> ()  [unwired: 1 out]
    n115 = global read "采配水全局变量.vi" "参数设置"() -> (w163:T10)
    n116 = global read "采配水全局变量.vi" "报警簇"() -> (w179:bool[])
    n117 = Enqueue Element(queue=w193, element=cluster{"命令":string, "数据":variant} {"命令"="读状态", "数据"=variant} ("元素")) -> (queue out=w175:refnum<queue>)  [unwired: 2 in, 2 out]
    n118 = Unbundle By Name(w191) -> ("R0"=w173:i16, "R1"=→"R1":i16, "R2"=→"R2":i16, "R12"=→"R12":i16, "R13"=→"R13":i16, "R14"=→"R14":i16, "R15"=→"R15":i16, "R16"=→"R16":i16, "R17"=→"R17":i16, "R18"=→"R18":i16, "R19"=→"R19":i16, "R20"=→"R20":i16, "R21"=→"R21":i16, "R22"=→"R22":i16, "R23"=→"R23":i16, "R24"=→"R24":i16, "R25"=→"R25":i16, "R26"=→"当前启动泵号":i16, "R33"=→"R33":i16)  [unwired: 9 out]
    "多列列表框" <- w173
    n119 = Unbundle By Name(w163) -> ("R117"=→"R117":i16)
    n120 = call "报警信息.vi"("报警簇"=w179) -> ("采配水报警信息"=w172:string)  [unwired: 9 in, 1 out]
    n121 = case shown="默认" w172 {
      selector: w172 -> [w195 _]
      tunnel: [w195 w196] -> w178
      frame Default {
      }
      frame "" {
        n122 = global read "采配水全局变量.vi" "运行状态显示"() -> (w196:string)
      }
    }
    "集成报警信息" <- w178
    n123 = Enqueue Element(queue=w175, element=cluster{"命令":string, "数据":variant} {"命令"="读参数", "数据"=variant} ("元素")) -> ()  [unwired: 2 in, 3 out]
    n124 = feedback-in #1(w173) -> ()
    n125 = feedback #1(w173) -> (w174:i16)
    n126 = Not Equal?(x=w174, y=w173) -> (x != y?=w180:bool)
    n127 = case shown="真" w180 {
      tunnel: w173 -> [_ w199]
      frame False {
      }
      frame True {
        n128 = property on="多列列表框" class="MCListbox (严格)"() -> ("ItemNames"=w200:string[][])  [unwired: 2 in, 2 out]
        n129 = Index Array(array=w200, index (row)=w199) -> (element=w198:string[])  [unwired: 1 in]
        n130 = Index Array(array=w198) -> (element=w197:string)  [unwired: 1 in]
        n131 = case shown="默认" w197 {
          selector: w197 -> [_ w201]
          frame "待机" {
          }
          frame Default {
            n132 = case shown="默认" w201 {
              selector: w201 -> [w207 _ _]
              tunnel: [w207 "-->>启动" "-->>结束"] -> w203
              frame Default {
              }
              frame "初始化" {
              }
              frame "结束" {
              }
            }
            n133 = Get Date/Time In Seconds() -> (seconds since 1Jan1904=w206:timestamp)
            n134 = Bundle("seconds since 1Jan1904"=w206, "table输入"="采配水", w203, "table输入"="") -> (w202:T11)  [unwired: 1 in]
            n135 = call "操作日志数据插入.vi"("data"=w202) -> ()  [unwired: 9 in, 1 out]
          }
        }
      }
    }
  }
  n136 = while {
    tunnel: w10 -> [w214]
    tunnel: w12 -> [w213]
    shift-right: [w217] -> w7
    shift-left: refnum<class "MB_Master.lvclass"> refnum ("MB session in") -> [w216]
    tunnel: errorcluster {"status"=FALSE, "code"=0, "source"=""} ("error out") -> [w215]
    tunnel: [w212] -> w8
    stop <- FALSE stop-if-true
    n137 = case shown="无错误" w215 {
      selector: w215 -> [w222 w384]
      tunnel: [w225 w383] -> w217
      tunnel: w216 -> [w224 w385]
      tunnel: [w223 w381] -> w212
      tunnel: w214 -> [w220 w380]
      tunnel: w213 -> [w219 _]
      frame No Error {
        n138 = Dequeue Element(queue=w220, error in (no error)=w219) -> (element=w218:cluster{"命令":string, "数据":variant})  [unwired: 1 in, 3 out]
        n139 = Unbundle By Name(w218) -> ("命令"=w221:string)
        n140 = case shown="\"读状态\"" w221 {
          tunnel: [w227 w228 w254 w335 w347 w357 w367 w376] -> w225
          tunnel: w224 -> [w227 w242 w305 w340 w350 w360 w370 w379]
          tunnel: [w226 w241 w252 w334 w348 w358 w368 w371] -> w223
          tunnel: w222 -> [w226 w244 w308 w339 w349 w359 w369 w377]
          tunnel: w218 -> [_ _ _ _ w346 w356 w366 _]
          frame "idle", Default {
          }
          frame "init" {
            w233 = refnum<visa-resource-name> "COM3" ("VISA resource name")
            n141 = call-dynamic "Close Session.vi"("error in (no error)"=w244, "MB session in"=w242) -> ("error out"=w243:errorcluster)  [unwired: 9 in]
            n142 = call <vilib>:"Clear Errors.vi"("error in (no error)"=w243) -> ("error out"=w231:errorcluster)  [unwired: 5 in, 1 out]
            n143 = call-poly "VISA Configure Serial Port"("VISA resource name"=w233, "baud rate (9600)"=u32 115200, "error in (no error)"=w231) -> ("VISA resource name out"=w235:refnum<visa-resource-name>, "error out"=w237:errorcluster)  [unwired: 11 in]
            n144 = VISA Write(VISA resource name=w235, write buffer="\u0002004701R04047560A5B\u0003" ("写入缓冲区"), error in (no error)=w237) -> (VISA resource name out=w234:refnum<visa-resource-name>, error out=w236:errorcluster)  [unwired: 1 out]
            n145 = VISA Close(VISA resource name=w234, error in (no error)=w236) -> (error out=w230:errorcluster)
            n146 = call <vilib>:"Open Serial Session.vi"("Mode (RTU)"=enum16{"RTU", "ASCII"}."RTU", "Error in"=w230, "Slave ID"=u8 10, "Serial Config"=T12 {"baud rate (bps)"=115200, "stop bits"=10, "parity"=0, "flow control"=0, "timeout"=500, "retries"=1}, "VISA Resource"=w233) -> ("Error out"=w241:errorcluster, "MB_Serial session"=w228:refnum<class "MB_Master_Serial.lvclass">)  [unwired: 5 in]
            n147 = Unbundle By Name(w241) -> ("status"=w245:bool)
            n148 = call "对话框信息"("Enable"=w245) -> ()  [unwired: 9 in, 2 out]
            n149 = global write "采配水全局变量.vi" "MB session in"(w228) -> ()
          }
          frame "读状态" {
            n150 = call <vilib>:"Read Holding Registers.vi"("error in (no error)"=w308, "quantity"=u16 80 ("number of holding registers"), "starting address"=u16 0, "MB session in"=w305) -> ("error out"=w303:errorcluster, "Registers"=w246:u16[], "MB session out"=w304:refnum<class "MB_Master.lvclass">)  [unwired: 5 in]
            "Registers" <- w246
            n151 = Array Subset(array=w246, index=27 ("索引")) -> (w273:u16[])  [unwired: 1 in]
            n152 = call <vilib>:"Read Holding Registers.vi"("error in (no error)"=w303, "quantity"=u16 6 ("number of holding registers"), "starting address"=u16 3840, "MB session in"=w304) -> ("error out"=w299:errorcluster, "Registers"=w276:u16[], "MB session out"=w300:refnum<class "MB_Master.lvclass">)  [unwired: 5 in]
            n153 = Array To Cluster(array=w246) -> (cluster=w247:T16)
            n154 = global write "采配水全局变量.vi" "状态"(w247) -> ()
            n155 = To Word Integer(number=w276) -> (16bit integer=w275:i16[])
            n156 = Array To Cluster(array=w276) -> (cluster=w316:T17)
            n157 = global write "采配水全局变量.vi" "AD"(w316) -> ()
            n158 = formula code="float AD0,AD1,AD2,AD3,AD4,AD5,AD6;\nAD0 = IN[0]*140/6553-75;\nAD1 = IN[1]/65.53-25;\nAD2 = IN[2]*30/8191;\nAD3 = IN[3]*30/8191;\nAD4 = IN[4]*30/8191;\nAD5 = IN[5]*30/8191;"("IN"=w275) -> ("AD0"=w314:dbl, "AD1"=w313:dbl, "AD2"=w312:dbl, "AD3"=w311:dbl, "AD4"=w310:dbl, "AD5"=w309:dbl)
            n159 = call <vilib>:"Read Coils.vi"("error in (no error)"=w299, "quantity"=u16 32 ("number of coils"), "starting address"=u16 0, "MB session in"=w300) -> ("error out"=w295:errorcluster, "Coils"=w280:bool[], "MB session out"=w296:refnum<class "MB_Master.lvclass">)  [unwired: 5 in]
            n160 = call "FATEK_HexToString.vi"("数组"=w273) -> ("STRING"=w272:string[])  [unwired: 10 in]
            n161 = global write "采配水全局变量.vi" "输出状态"(w280) -> ()
            n162 = Index Array(array=w272) -> (element=→"采配水版本号":string)  [unwired: 1 in]
            n163 = Bundle(w314, w313, w312, w311, w310, w309) -> (w315:cluster{dbl, dbl, dbl, dbl, dbl, dbl})  [unwired: 1 in]
            n164 = Index Array(array=w280, index #7=13 ("索引")) -> (element #1=w270:bool, element #2=w269:bool, element #3=w268:bool, element #4=w267:bool, element #5=w266:bool, element #6=w265:bool, element #7=w263:bool, element #8=w262:bool, element #11=w261:bool, element #12=w260:bool, element #14=w256:bool)  [unwired: 13 in, 3 out]
            n165 = global write "采配水全局变量.vi" "转换值"(w315) -> ()
            n166 = call <vilib>:"Read Coils.vi"("error in (no error)"=w295, "quantity"=u16 16 ("number of coils"), "starting address"=u16 1000, "MB session in"=w296) -> ("error out"=w291:errorcluster, "Coils"=w287:bool[], "MB session out"=w292:refnum<class "MB_Master.lvclass">)  [unwired: 5 in]
            n167 = local write "V1"(w270) -> ()
            n168 = local write "V2"(w269) -> ()
            n169 = local write "V3"(w268) -> ()
            n170 = local write "V4"(w267) -> ()
            n171 = local write "V5"(w266) -> ()
            n172 = local write "V6"(w265) -> ()
            n173 = local write "M1-1"(w261) -> ()
            n174 = local write "M1-2"(w260) -> ()
            n175 = local write "M2"(w256) -> ()
            n176 = global write "采配水全局变量.vi" "输入状态"(w287) -> ()
            n177 = Index Array(array=w287) -> (element #1=→"X0":bool, element #2=→"X1":bool, element #3=→"X2":bool, element #4=→"X3":bool, element #5=→"X4":bool, element #6=→"X5":bool, element #7=→"X6":bool, element #8=→"X7":bool, element #9=→"X8":bool, element #10=→"X9":bool, element #11=→"X10":bool, element #12=→"X11":bool)  [unwired: 12 in]
            n178 = local write "V13NO"(w263) -> ()
            n179 = local write "V13NC"(w262) -> ()
            n180 = call <vilib>:"Read Coils.vi"("error in (no error)"=w291, "quantity"=u16 16 ("number of coils"), "starting address"=u16 2500, "MB session in"=w292) -> ("error out"=w253:errorcluster, "Coils"=w288:bool[], "MB session out"=w255:refnum<class "MB_Master.lvclass">)  [unwired: 5 in]
            n181 = global write "采配水全局变量.vi" "报警簇"(w288) -> ()
            n182 = call <vilib>:"Read Coils.vi"("error in (no error)"=w253, "quantity"=u16 1 ("starting address"), "starting address"=u16 2801, "MB session in"=w255) -> ("error out"=w252:errorcluster, "Coils"=w249:bool[], "MB session out"=w254:refnum<class "MB_Master.lvclass">)  [unwired: 5 in]
            n183 = Index Array(array=w249) -> (element=w248:bool)  [unwired: 1 in]
            n184 = local write "看门狗启用"(w248) -> ()
          }
          frame "读参数" {
            n185 = call <vilib>:"Read Holding Registers.vi"("error in (no error)"=w339, "quantity"=u16 20 ("number of holding registers"), "starting address"=u16 100, "MB session in"=w340) -> ("error out"=w334:errorcluster, "Registers"=w336:u16[], "MB session out"=w335:refnum<class "MB_Master.lvclass">)  [unwired: 5 in]
            n186 = Array To Cluster(array=w336) -> (cluster=w323:T18)
            n187 = global write "采配水全局变量.vi" "参数设置"(w323) -> ()
            n188 = Unbundle(w323) -> ("Registers[0]"=→"R100":u16, "Registers[1]"=→"R101":u16, "Registers[2]"=→"R102":u16, "Registers[3]"=→"R103":u16, "Registers[4]"=→"R104":u16, "Registers[5]"=→"R105":u16, "Registers[6]"=→"R106":u16, "Registers[7]"=→"R107":u16, "Registers[8]"=→"R108":u16, "Registers[9]"=→"R109":u16, "Registers[10]"=w322:u16, "Registers[11]"=→"R111":u16, "Registers[12]"=→"R112":u16, "Registers[13]"=→"R113":u16, "Registers[16]"=w318:u16, "Registers[18]"=→"R118":u16)  [unwired: 18 out]
            n189 = local write "R116"(w318) -> ()
            n190 = local write "潜水泵工作模式"(w322) -> ()
          }
          frame "多个写入" {
            n191 = Unbundle By Name(w346) -> ("数据"=w345:variant)
            n192 = Variant To Data(type=T13 {"starting address"=0, "holding register values"=[]}, Variant=w345) -> (data=w343:T13)  [unwired: 1 in, 1 out]
            n193 = Unbundle By Name(w343) -> ("starting address"=w342:u16, "holding register values"=w341:u16[])
            n194 = call <vilib>:"Write Multiple Registers.vi"("error in (no error)"=w349, "values"=w341, "starting address"=w342, "MB session in"=w350) -> ("error out"=w348:errorcluster, "MB session out"=w347:refnum<class "MB_Master.lvclass">)  [unwired: 6 in]
          }
          frame "单个写入" {
            n195 = Unbundle By Name(w356) -> ("数据"=w355:variant)
            n196 = Variant To Data(type=T14 {"starting address"=0, "holding register value"=0}, Variant=w355) -> (data=w353:T14)  [unwired: 1 in, 1 out]
            n197 = Unbundle By Name(w353) -> ("starting address"=w352:u16, "holding register value"=w351:u16)
            n198 = call <vilib>:"Write Single Register.vi"("error in (no error)"=w359, "value"=w351, "address"=w352, "MB session in"=w360) -> ("error out"=w358:errorcluster, "MB session out"=w357:refnum<class "MB_Master.lvclass">)  [unwired: 6 in]
          }
          frame "线圈写入" {
            n199 = Unbundle By Name(w366) -> ("数据"=w365:variant)
            n200 = Variant To Data(type=T15 {"starting address"=0, "coil values"=[]}, Variant=w365) -> (data=w363:T15)  [unwired: 1 in, 1 out]
            n201 = Unbundle By Name(w363) -> ("starting address"=w362:u16, "coil values"=w361:bool[])
            n202 = call <vilib>:"Write Multiple Coils.vi"("error in (no error)"=w369, "values"=w361, "starting address"=w362, "MB session in"=w370) -> ("error out"=w368:errorcluster, "MB session out"=w367:refnum<class "MB_Master.lvclass">)  [unwired: 6 in]
          }
          frame "shutdown" {
            n203 = call <vilib>:"Write Single Register.vi"("error in (no error)"=w377, "value"=u16 0, "address"=u16 4047, "MB session in"=w379) -> ("error out"=w378:errorcluster, "MB session out"=w376:refnum<class "MB_Master.lvclass">)  [unwired: 6 in]
            n204 = call-dynamic "Close Session.vi"("error in (no error)"=w378, "MB session in"=w376) -> ("error out"=w372:errorcluster)  [unwired: 9 in]
            n205 = call <vilib>:"Clear Errors.vi"("error in (no error)"=w372) -> ("error out"=w373:errorcluster)  [unwired: 5 in, 1 out]
            n206 = call "调用WinProladder.vi"("错误输入（无错误）"=w373) -> ("错误输出"=w371:errorcluster)  [unwired: 10 in]
          }
        }
      }
      frame Error {
        n207 = Unbundle By Name(w384) -> ("code"=w386:i32)
        n208 = case shown="-1073807343" w386 {
          tunnel: w385 -> [w388 w392]
          tunnel: w384 -> [w387 w394]
          tunnel: [w387 w393] -> w382
          tunnel: [w388 w392] -> w383
          tunnel: w380 -> [_ w391]
          frame Default {
          }
          frame -1073807343 {
            n209 = Flush Queue(queue=w391) -> (queue out=w390:refnum<queue>)  [unwired: 1 in, 2 out]
            n210 = call-dynamic "Close Session.vi"("error in (no error)"=w394, "MB session in"=w392) -> ("error out"=w393:errorcluster)  [unwired: 9 in]
            n211 = disable-structure shown="禁用" {
              disable-tunnel: w390 -> [w395 _]
              frame Disabled {
                n212 = Enqueue Element At Opposite End(queue=w395, element=cluster{"命令":string, "数据":variant} {"命令"="init", "数据"=variant} ("元素")) -> ()  [unwired: 2 in, 3 out]
              }
              frame Enabled {
              }
            }
            n213 = Wait (ms)(milliseconds to wait=u32 2000 ("等待时间（毫秒）")) -> ()  [unwired: 1 out]
          }
        }
        n214 = call <vilib>:"Clear Errors.vi"("error in (no error)"=w382) -> ("error out"=w381:errorcluster)  [unwired: 5 in, 1 out]
      }
    }
    n215 = Unbundle By Name(w212) -> ("status"=→"通讯故障":bool)
  }
  n216 = property on="多列列表框" class="MCListbox (严格)"("ItemNames"=string[][] [["待机"], ["初始化"], ["外部管路润洗"], ["内部管路润洗"], ["采样"], ["沉淀"], ["配水"], ["外部管路反冲洗"], ["内部管路反冲洗"], ["采样池储水"], ["结束"]] ("项名")) -> ()  [unwired: 2 in, 2 out]
  n217 = call-dynamic "Close Session.vi"("error in (no error)"=w8, "MB session in"=w7) -> ()  [unwired: 9 in, 1 out]
